vi "GetFirstScreen.vi"(8 "error in (no error)":errorcluster, 11 "SnakeGame in":refnum<class "SnakeGame.lvclass">) -> (0 "error out":errorcluster, 2 "Array":u32[][](array[numeric]), 3 "SnakeGame out":refnum<class "SnakeGame.lvclass">)   [LabVIEW 2019, in "RT_Game.lvlib" / "SnakeGame.lvclass"]
uses:
  SnakeGame.lvclass
  C:/Users/FreshBob/Dropbox/VIs/myRIO_GameConsole/RT/RT_Game/Game/Game.lvclass
  Game/Game.lvclass/Game.ctl
  Game/Read Singleplayer.vi
  Game/Game.lvclass
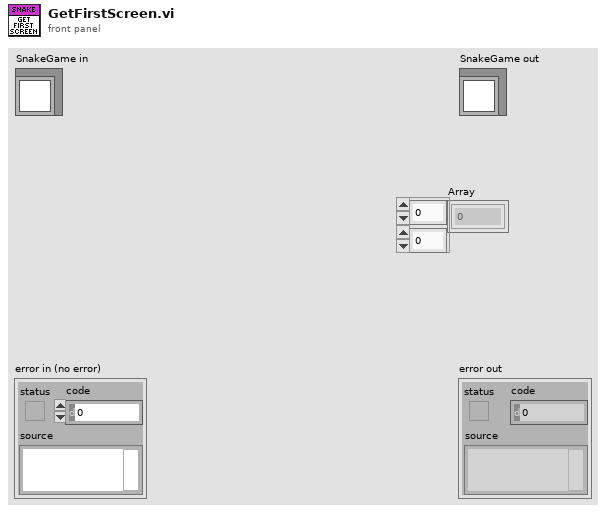
[diagram p1: front panel]
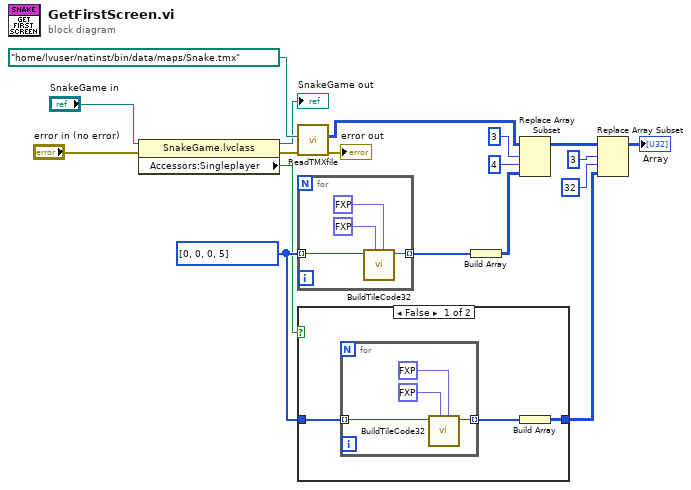
[diagram p0: block diagram]
diagram:
  w5 = u32[] [0, 0, 0, 5]
  n1 = property class="SnakeGame.lvclass"(reference="SnakeGame in", error in="error in (no error)") -> (reference out=→"SnakeGame out":refnum<class "SnakeGame.lvclass">, error out=w4:errorcluster, "Accessors:Singleplayer"=w1:bool)
  n2 = call "ReadTMXfile.vi"("error in (no error)"=w4, "path to tmx-file (created with Tiles2D)"=path "/home/lvuser/natinst/bin/data/maps/Snake.tmx") -> ("error out"=→"error out":errorcluster, "Tilenumbers"=w15:u32[][])  [unwired: 8 in]
  n3 = for {
    tunnel: [w22] -> w6 mode=indexing
    tunnel: w5 -> [w19] mode=indexing
    n4 = call "BuildTileCode32.vi"("replacecolor"=fxp<+,3,3> 1.0, "color_to_replace"=fxp<+,3,3> 7.0, "Tilenumber"=w19) -> ("TileCode"=w22:u32)  [unwired: 8 in]
  }
  n5 = case shown="False" w1 {
    tunnel: [w25 _] -> w7
    tunnel: w5 -> [w23 _]
    frame False {
      n6 = for {
        tunnel: w23 -> [w29] mode=indexing
        tunnel: [w26] -> w24 mode=indexing
        n7 = call "BuildTileCode32.vi"("replacecolor"=fxp<+,3,3> 2.0, "color_to_replace"=fxp<+,3,3> 7.0, "Tilenumber"=w29) -> ("TileCode"=w26:u32)  [unwired: 8 in]
      }
      n8 = Build Array(w24) -> (w25:u32[][])
    }
    frame True {
    }
  }
  n9 = Build Array(w6) -> (w11:u32[][])
  n10 = Replace Array Subset(array=w15, new element=w11, index (row)=3, index (col)=4 ("disabled index (col)")) -> (w14:u32[][])
  n11 = Replace Array Subset(array=w14, new element=w7, index (row)=3, index (col)=32 ("disabled index (col)")) -> (→"Array":u32[][])
